vi "Load Configuration Tool.vi"() -> ()   [LabVIEW 2013]
uses:
  NationalInstruments.VeriStand.SystemStorageUI
  NationalInstruments.VeriStand.SystemStorage
  <vilib>/NI Veristand/Execution/Workspace/NI VeriStand - Set Multiple Channel Values.vi
  <vilib>/NI Veristand/Execution/Workspace/NI_VS Workspace ExecutionAPI.lvlib
  <vilib>/NI Veristand/UI Controls/Single Node Browser/NI_VS UI Single Node Browser.lvlib
  MUX Custom Device.lvlib
panel:
  in  "Cancel":bool
  in  "OK":bool
  in  "MUX Configuration Path":path
  in  "NIVS.System Definition Root":refnum<k24>
  in  "PXI-2569 MUX":refnum<k24>(container)
  in  "NIVS.Workspace Event":refnum<event-registration>
  out "Targets":string[](array[string])
  in  "NIVS.Gateway IP Address":string
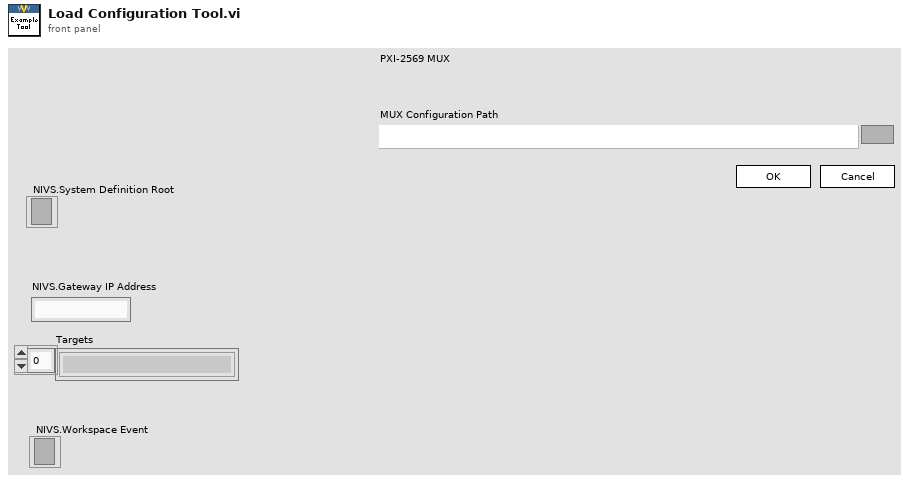
[diagram p1: front panel]
types:
  T1 = typedef "NI_VS UI Single Node Browser.lvlib/Callback Type.ctl" = cluster{"Net Callbacks":refnum<k27>[], "Event":refnum<user-event>}
  T2 = typedef "NI_VS Workspace ExecutionAPI.lvlib/WorkspaceAPI.ctl" = refnum<k24>
  T3 = typedef "NI_VS Workspace ExecutionAPI.lvlib/SystemStateEventRef.ctl" = cluster{"CustDatRef":refnum<user-event>, "EvtRef":refnum<k27>}
  T4 = typedef "NI_VS Workspace ExecutionAPI.lvlib/SystemStateRegEventRef.ctl" = refnum<event-registration>
  T5 = cluster{"NIVS.Workspace Event":refnum<event-registration>, "Event Registration Refnum":refnum<event-registration>, "SystemChangeEventRef":T4}
  T6 = enum8{"Enabled", "Disabled", "Disabled and Grayed Out"}
  T7 = typedef "NI_VS Workspace ExecutionAPI.lvlib/SystemState.ctl" = u8
  T8 = typedef "MUX Custom Device.lvlib/Mux Data.ctl" = cluster{"Mux Name":string, "Relay Channel Data":T9[]}
  T9 = typedef "MUX Custom Device.lvlib/Relay Channel Data.ctl" = cluster{"Relay Channel Name":string, "Relay Data":T10}
  T10 = typedef "MUX Custom Device.lvlib/Relay Data.ctl" = cluster{"Relay Name":string, "State":T11}
  T11 = typedef "MUX Custom Device.lvlib/Switch.ctl" = bool
  T12 = typedef "NI_VS UI Single Node Browser.lvlib/Node Ref.ctl" = refnum<k24>
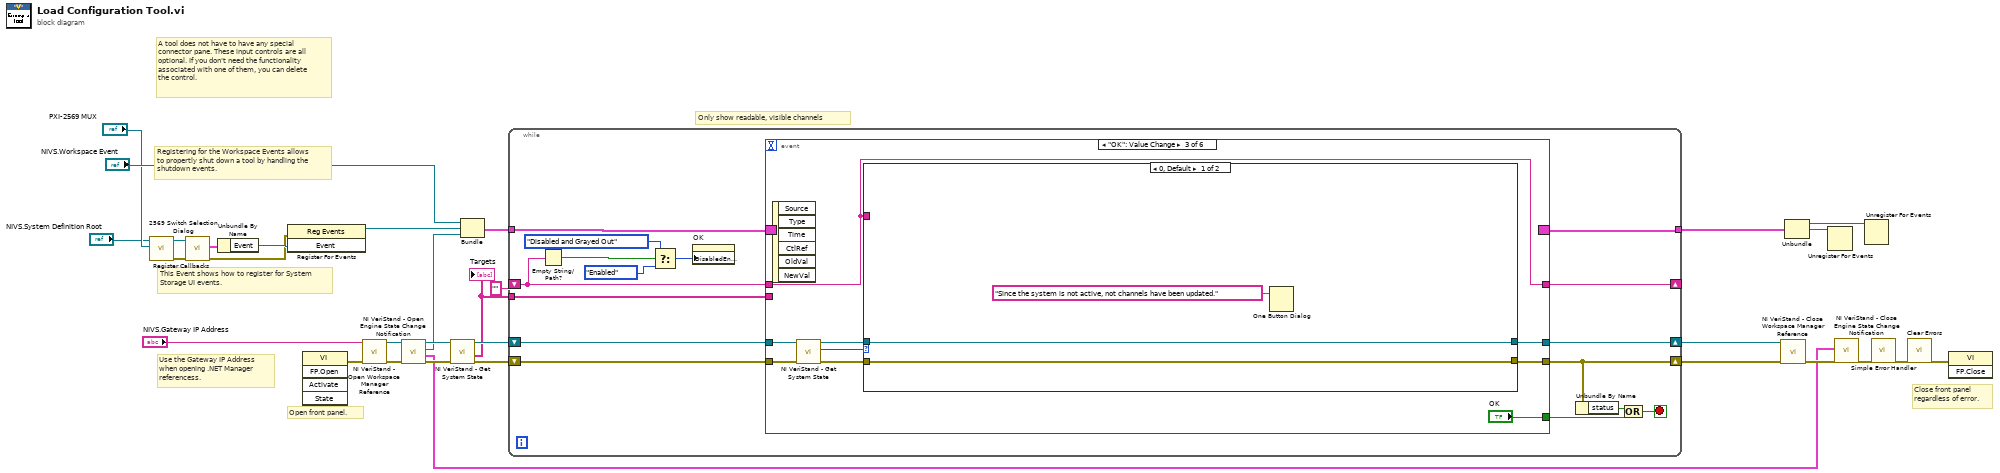
[diagram p0: block diagram]
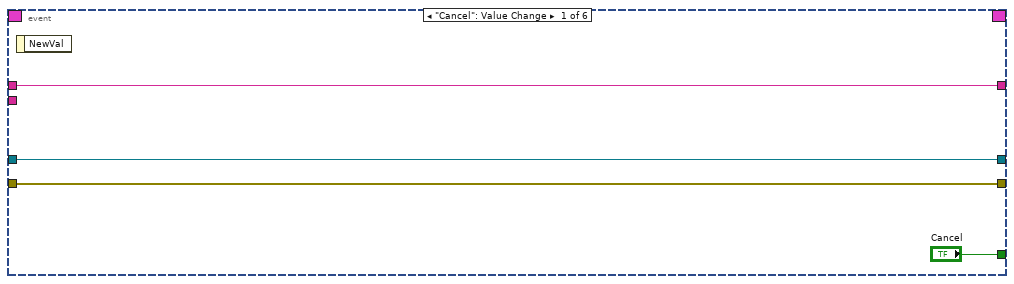
[diagram p2: hidden frame]
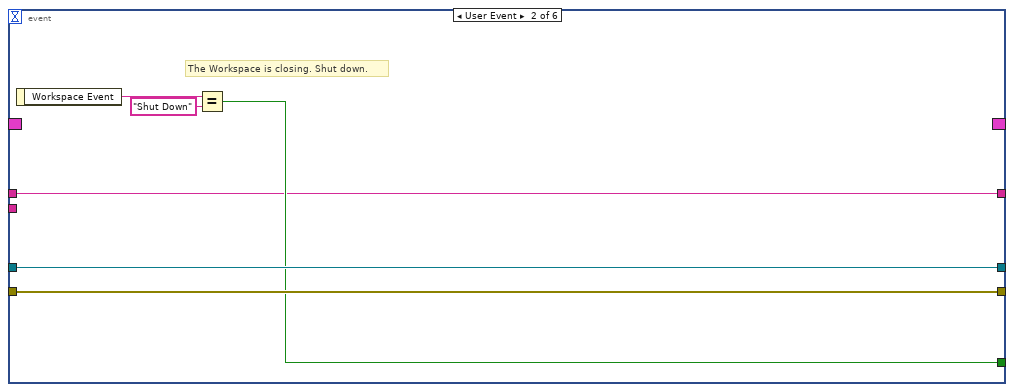
[diagram p3: hidden frame]
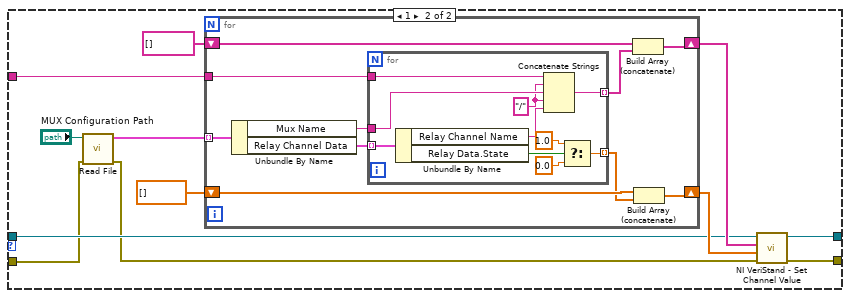
[diagram p4: hidden frame]
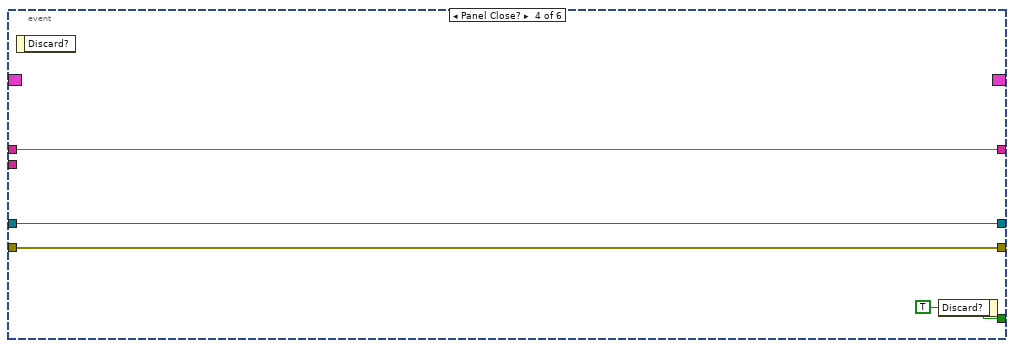
[diagram p5: hidden frame]
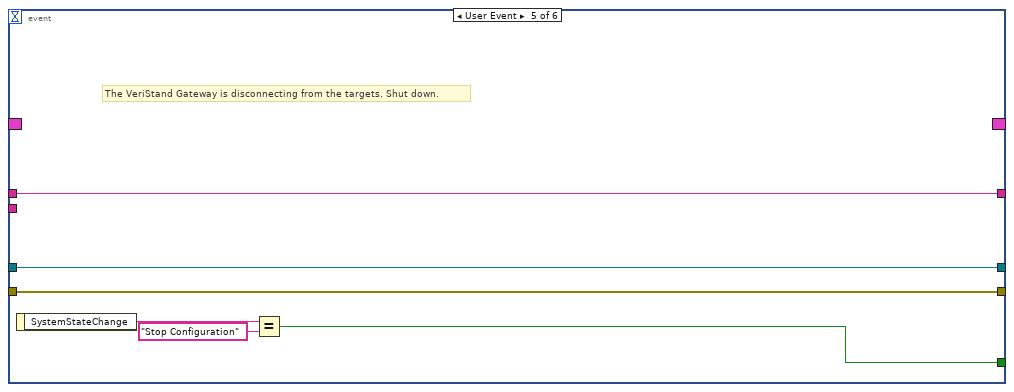
[diagram p6: hidden frame]
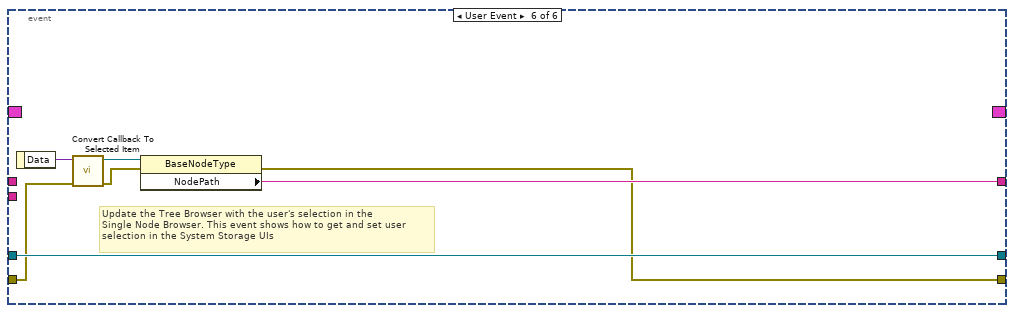
[diagram p7: hidden frame]
diagram:
  # "Only show readable, visible channels"
  # "This Event shows how to register for System Storage UI events."
  # "Use the Gateway IP Address when opening .NET Manager referencess."
  # "A tool does not have to have any special connector pane. These input controls are all optional. If you don't need the functionality associated with one of them, you can delete the control."
  # "Registering for the Workspace Events allows to propertly shut down a tool by handling the shutdown events."
  # "Close front panel\nregardless of error."
  # "Open front panel."
  n1 = call "2569 Switch Selection Dialog.vi"("NodeBroswerWF in"="PXI-2569 MUX", "NIVS.System Definition Root"="NIVS.System Definition Root") -> ("error out"=w4:errorcluster, "NodeBrowserWF out"=w3:refnum<k24>)  [unwired: 8 in]
  n2 = call <vilib>:"Register Callbacks.vi"("error in (no error)"=w4, "Single Node Browser"=w3) -> ("error out"=w6:errorcluster, "Callbacks"=w8:T1)  [unwired: 7 in, 1 out]
  n3 = Unbundle By Name(w8) -> ("Event"=w7:refnum<user-event>)
  n4 = register-events(error in=w6, w7) -> (reference out=w10:refnum<event-registration>)  [unwired: 1 in, 1 out]
  n5 = invoke class="VI" method="FP.Open"() -> (error out=w14:errorcluster)  [unwired: 5 in, 4 out]
  n6 = call <vilib>:"NI VeriStand - Open Workspace Manager Reference.vi"("error in (no error)"=w14, "Gateway IP Address (\"\": localhost)"="NIVS.Gateway IP Address") -> ("error out"=w25:errorcluster, "WorkspaceManager"=w26:T2)  [unwired: 8 in]
  n7 = call <vilib>:"NI VeriStand - Open Engine State Change Notification.vi"("error in (no error)"=w25, "WorkspaceManager in"=w26) -> ("error out"=w30:errorcluster, "SystemStateRefs"=w19:T3, "SystemChangeEventRef"=w9:T4, "WorkspaceManager out"=w31:T2)  [unwired: 6 in]
  n8 = call <vilib>:"NI VeriStand - Get System State.vi"("error in (no error)"=w30, "WorkspaceManager in"=w31) -> ("error out"=w17:errorcluster, "Targets"=w16:string[], "WorkspaceManager  out"=w18:T2)  [unwired: 5 in, 2 out]
  "Targets" <- w16
  n9 = Bundle("NIVS.Workspace Event"="NIVS.Workspace Event", "Event Registration Refnum"=w10, "SystemChangeEventRef"=w9) -> (w24:T5)  [unwired: 1 in]
  n10 = while {
    tunnel: w24 -> [w47]
    tunnel: [w46] -> w23
    shift-right: [w40] -> w27
    shift-left: w17 -> [w44]
    shift-right: [w43] -> w28
    shift-left: w18 -> [w45]
    tunnel: w16 -> [w42]
    shift-right: [w37] -> _
    shift-left: "" ("NodePath") -> [w36]
    stop <- w38 stop-if-true
    n11 = Empty String/Path?(string/path=w36) -> (empty?=w33:bool)
    n12 = Select(t=T6."Disabled and Grayed Out" ("Disabled"), s=w33, f=T6."Enabled" ("Disabled")) -> (s? t:f=w32:T6)
    n13 = property on="OK" class="Bool"("DisabledEnum"=w32) -> ()  [unwired: 2 in, 2 out]
    n14 = event shown="[2] \"OK\": Value Change" {
      selector: w47 -> [_ _ _ _ _ _]
      dyn-events: [_ _ _ _ _ _] -> w46
      timeout: _ -> [_ _ _ _ _ _]
      tunnel: ["Cancel" w53 "OK" w103 w107 _] -> w39
      tunnel: w45 -> [w50 w56 w61 w104 w110 w118]
      tunnel: w44 -> [w51 w57 w62 w105 w111 w116]
      tunnel: [w51 w57 w64 w105 w111 w112] -> w40
      tunnel: [w50 w56 w65 w104 w110 w118] -> w43
      tunnel: w42 -> [_ _ _ _ _ _]
      tunnel: [w49 w52 w63 w102 w106 w113] -> w37
      tunnel: w36 -> [w49 w52 w63 w102 w106 _]
      event "Cancel": Value Change {
        n15 = event-data() -> ()  [unwired: 1 in, 1 out]
      }
      event User Event {
        # "The Workspace is closing. Shut down."
        n16 = event-data() -> ("Workspace Event"=w55:string)  [unwired: 1 in]
        n17 = Equal?(x=w55, y="Shut Down") -> (x = y?=w53:bool)
      }
      event "OK": Value Change {
        n18 = event-data() -> ()  [unwired: 1 in, 6 out]
        n19 = call <vilib>:"NI VeriStand - Get System State.vi"("error in (no error)"=w62, "WorkspaceManager in"=w61) -> ("error out"=w59:errorcluster, "System State"=w58:T7, "WorkspaceManager  out"=w60:T2)  [unwired: 5 in, 2 out]
        n20 = case shown="0, Default" w58 {
          tunnel: w60 -> [w68 w75]
          tunnel: [w68 w74] -> w65
          tunnel: [w69 w73] -> w64
          tunnel: w63 -> [_ w72]
          tunnel: w59 -> [w69 w71]
          frame 0, Default {
            n21 = One Button Dialog(message="Since the system is not active, not channels have been updated.") -> ()  [unwired: 1 in, 1 out]
          }
          frame 1 {
            n22 = call "Read File.vi"("Error In"=w71, "Mux File Path"="MUX Configuration Path") -> ("Error Out"=w70:errorcluster, "Mux Data Array"=w81:T8[])  [unwired: 8 in]
            n23 = for {
              tunnel: w81 -> [w91] mode=indexing
              tunnel: w72 -> [w89]
              shift-right: [w85] -> w78
              shift-left: string[] [] -> [w87]
              shift-right: [w82] -> w76
              shift-left: dbl[] [] -> [w84]
              n24 = Unbundle By Name(w91) -> ("Mux Name"=w88:string, "Relay Channel Data"=w90:T9[])
              n25 = for {
                tunnel: w90 -> [w101] mode=indexing
                tunnel: w89 -> [w100]
                tunnel: w88 -> [w99]
                tunnel: [w93] -> w83 mode=indexing
                tunnel: [w92] -> w86 mode=indexing
                w98 = "/" ("string")
                n26 = Unbundle By Name(w101) -> ("Relay Channel Name"=w97:string, "Relay Data.State"=w94:T11)
                n27 = Concatenate Strings(w100, w98, w99, w98, w97) -> (w92:string)
                n28 = Select(t=1.0, s=w94, f=0.0) -> (s? t:f=w93:dbl)
              }
              n29 = Build Array (concatenate)(w87, w86) -> (w85:string[])
              n30 = Build Array (concatenate)(w84, w83) -> (w82:dbl[])
            }
            n31 = call-poly <vilib>:"NI VeriStand - Set Channel Value.vi"("error in (no error)"=w70, "Values"=w76, "Channels"=w78, "WorkspaceManager in"=w75) -> ("error out"=w73:errorcluster, "WorkspaceManager out"=w74:T2)  [unwired: 6 in]
          }
        }
      }
      event Panel Close? {
        w103 = TRUE ("Discard?")
        n32 = event-data() -> ()  [unwired: 1 in, 1 out]
        n33 = event-data("Discard?"=w103) -> ()  [unwired: 1 in, 1 out]
      }
      event User Event {
        # "The VeriStand Gateway is disconnecting from the targets. Shut down."
        n34 = event-data() -> ("SystemStateChange"=w109:string)  [unwired: 1 in]
        n35 = Equal?(x=w109, y="Stop Configuration") -> (x = y?=w107:bool)
      }
      event User Event {
        # "Update the Tree Browser with the user's selection in the\nSingle Node Browser. This event shows how to get and set user\nselection in the System Storage UIs"
        n36 = event-data() -> ("Data"=w117:variant)  [unwired: 1 in]
        n37 = call <vilib>:"Convert Callback To Selected Item.vi"("error in"=w116, "Data"=w117) -> ("error out"=w114:errorcluster, "Selected Item"=w115:T12)  [unwired: 8 in]
        n38 = property class="BaseNodeType"(reference=w115, error in=w114) -> (error out=w112:errorcluster, "NodePath"=w113:string)  [unwired: 1 out]
      }
    }
    n39 = Unbundle By Name(w40) -> ("status"=w41:bool)
    n40 = Compound Arithmetic op=OR(w41, w39) -> (w38:bool)
  }
  n41 = call <vilib>:"NI VeriStand - Close Workspace Manager Reference.vi"("error in (no error)"=w27, "WorkspaceManager"=w28) -> ("error out"=w20:errorcluster)  [unwired: 9 in]
  n42 = Unbundle(w23) -> ("NIVS.Workspace Event"=w21:refnum<event-registration>, "Event Registration Refnum"=w22:refnum<event-registration>)  [unwired: 1 out]
  n43 = Unregister For Events(event registration refnum=w22) -> ()  [unwired: 1 in, 1 out]
  n44 = call <vilib>:"NI VeriStand - Close Engine State Change Notification.vi"("error in (no error)"=w20, "SystemStateRefs"=w19) -> ("error out"=w13:errorcluster)  [unwired: 9 in]
  n45 = Unregister For Events(event registration refnum=w21) -> ()  [unwired: 1 in, 1 out]
  n46 = call <vilib>:"Simple Error Handler.vi"("error in (no error)"=w13) -> ("error out"=w12:errorcluster)  [unwired: 4 in, 4 out]
  n47 = call <vilib>:"Clear Errors.vi"("error in (no error)"=w12) -> ("error out"=w11:errorcluster)  [unwired: 6 in]
  n48 = invoke class="VI" method="FP.Close"(error in=w11) -> ()  [unwired: 2 in, 3 out]
